vi "1D Quadrature (Formula).vi"(8 "tolerance":dbl=1e-05, 9 "lower limit":dbl, 10 "upper limit":dbl=1.0, 11 "integrand":string) -> (0 "error":i32, 3 "result":dbl)   [LabVIEW 2020, in "NI_AALPro.lvlib"]
doc: "Performs numerical integration using adaptive quadrature approach. You must manually select the polymorphic instance to use."
uses:
  <vilib>/Analysis/NI_AALPro.lvlib
panel:
  # "Use x as the independent variable in integrand.\nExample:\nintegrand:  sin(x)\nupper limit = 1, lower limit = 0,\nresult = 0.459698"
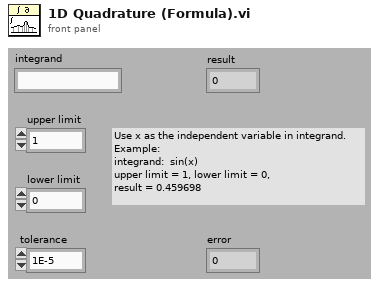
[diagram p1: front panel]
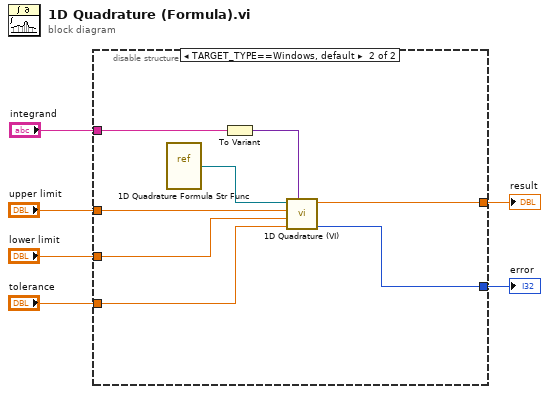
[diagram p0: block diagram]
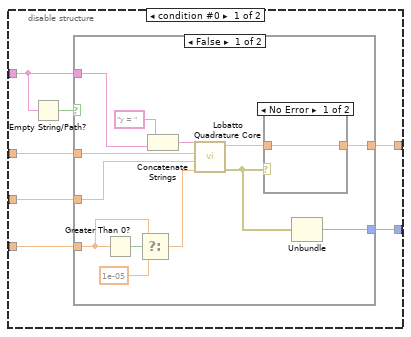
[diagram p2: hidden frame]
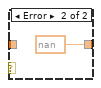
[diagram p3: hidden frame]
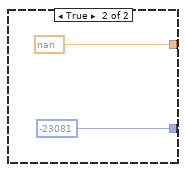
[diagram p4: hidden frame]
diagram:
  n1 = disable-structure shown="TARGET_TYPE==Windows, default" {
    disable-tunnel: [w12 w34] -> w6
    disable-tunnel: "integrand" -> [w11 w32]
    disable-tunnel: "upper limit" -> [w10 w38]
    disable-tunnel: "lower limit" -> [w9 w37]
    disable-tunnel: "tolerance" -> [w8 w36]
    disable-tunnel: [w7 w35] -> w1
    frame condition #0 {
      n2 = Empty String/Path?(string/path=w11) -> (empty?=w13:bool)
      n3 = case shown="False" w13 {
        tunnel: [w23 nan] -> w7
        tunnel: [w21 -23081] -> w12
        tunnel: w11 -> [w20 _]
        tunnel: w10 -> [w26 _]
        tunnel: w9 -> [w25 _]
        tunnel: w8 -> [w15 _]
        frame False {
          n4 = Greater Than 0?(x=w15) -> (x > 0?=w17:bool)
          n5 = Select(t=w15, s=w17, f=1e-05) -> (s? t:f=w14:dbl)
          n6 = Concatenate Strings("y = ", w20) -> (w18:string)
          n7 = call <vilib>:"Lobatto Quadrature Core.vi"("tolerance"=w14, "lower limit"=w25, "upper limit"=w26, "formula"=w18) -> ("error out"=w22:errorcluster, "result"=w24:dbl)  [unwired: 6 in]
          n8 = case shown="No Error" w22 {
            tunnel: w24 -> [w27 _]
            tunnel: [w27 nan] -> w23
            frame No Error {
            }
            frame Error {
            }
          }
          n9 = Unbundle(w22) -> ("code"=w21:i32)  [unwired: 2 out]
        }
        frame True {
        }
      }
    }
    frame condition #1 (active) {
      n10 = vi-ref <vilib>:"1D Quadrature Formula Str Func.vi"() -> (w31:refnum<vi>)
      n11 = To Variant(anything=w32) -> (Variant=w33:variant)
      n12 = call <vilib>:"1D Quadrature (VI).vi"("data"=w33, "tolerance"=w36, "lower limit"=w37, "upper limit"=w38, "integrand"=w31) -> ("error"=w34:i32, "result"=w35:dbl)  [unwired: 5 out]
    }
  }
  "error" <- w6
  "result" <- w1
